vi "Get Cluster Items.vi"(7 "Recursive?":bool=TRUE, 8 "Error in":errorcluster, 11 "Clust Refnum":refnum<vi>) -> (0 "Error out":errorcluster, 3 "Controls[]":refnum<vi>[](array[refnum]))   [LabVIEW 2021, in "EDT VIE.lvlib"]
uses:
  EDT VIE.lvlib
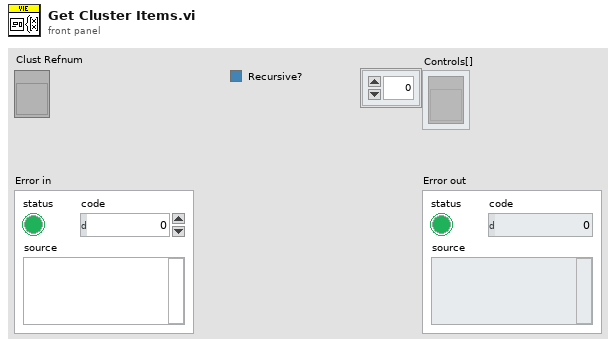
[diagram p1: front panel]
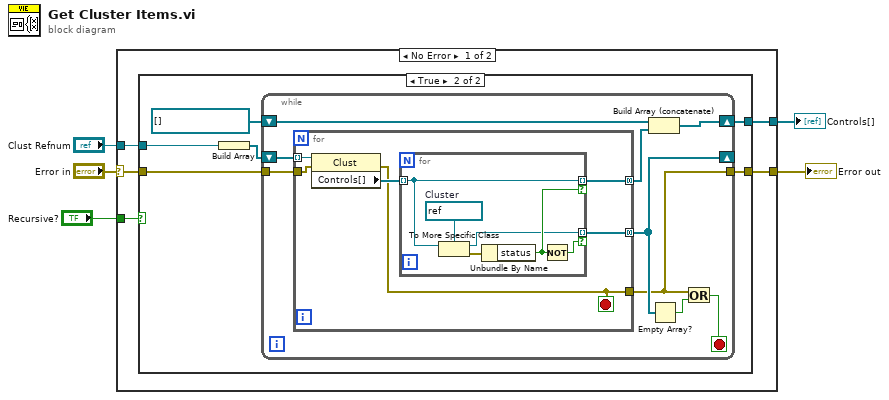
[diagram p0: block diagram]
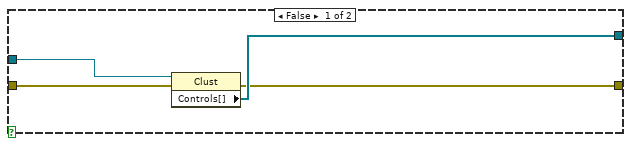
[diagram p2: hidden frame]
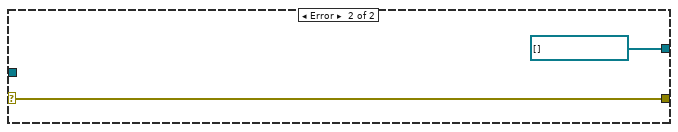
[diagram p3: hidden frame]
diagram:
  n1 = case shown="No Error" "Error in" {
    selector: "Error in" -> [w8 w42]
    tunnel: "Clust Refnum" -> [w10 _]
    tunnel: [w9 refnum<vi>[] [] ("Controls[]")] -> w4
    tunnel: [w7 w42] -> w2
    tunnel: "Recursive?" -> [w6 _]
    frame No Error {
      n2 = case shown="True" w6 {
        tunnel: w10 -> [w14 w20]
        tunnel: [w13 w17] -> w9
        tunnel: w8 -> [w12 w16]
        tunnel: [w11 w15] -> w7
        frame False {
          n3 = property class="Clust"(reference=w14, error in=w12) -> (error out=w11:errorcluster, "Controls[]"=w13:refnum<vi>[])  [unwired: 1 out]
        }
        frame True {
          n4 = Build Array(w20) -> (w18:refnum<vi>[])
          n5 = while {
            shift-right: [w25] -> w17
            shift-left: refnum<vi>[] [] ("Controls[]") -> [w26]
            shift-right: [w28] -> _
            shift-left: w18 -> [w29]
            tunnel: w16 -> [w24]
            tunnel: [w21] -> w15
            stop <- w22 stop-if-true
            n6 = for {
              tunnel: w29 -> [w35] mode=indexing
              tunnel: [w33] -> w28 mode=concatenating
              tunnel: [w32] -> w27 mode=concatenating
              tunnel: w24 -> [w31]
              tunnel: [w30] -> w21
              stop <- w30 stop-if-true
              n7 = property class="Clust"(reference=w35, error in=w31) -> (error out=w30:errorcluster, "Controls[]"=w34:refnum<vi>[])  [unwired: 1 out]
              n8 = for {
                tunnel: w34 -> [w37] mode=indexing
                tunnel: [w37] -> w32 mode=indexing if=w38
                tunnel: [w36] -> w33 mode=indexing if=w39
                w41 = refnum<vi> refnum  # Cluster
                n9 = To More Specific Class(target class=w41, reference=w37) -> (specific class reference=w36:refnum<vi>, error out=w40:errorcluster)  [unwired: 1 in]
                n10 = Unbundle By Name(w40) -> ("status"=w38:bool)
                n11 = Not(x=w38) -> (.not. x?=w39:bool)
              }
            }
            n12 = Build Array (concatenate)(w26, w27) -> (w25:refnum<vi>[])
            n13 = Empty Array?(array=w28) -> (empty?=w23:bool)
            n14 = Or(x=w21, y=w23) -> (x .or. y?=w22:bool)
          }
        }
      }
    }
    frame Error {
    }
  }
  "Controls[]" <- w4
  "Error out" <- w2
